vi "Transparent_VI.vi"(5 "Error_In":errorcluster) -> (19 "Error_Out":errorcluster)   [LabVIEW 2023]
doc: "Used to Popup in background for better UI and UX"
uses:
  Controls/UE_Driver_Operation_Select.ctl
types:
  T1 = typedef "UE_Driver_Operation_Select.ctl" = enum16{"Create_UE", "Get_Refnum", "Generate_UE", "Destroy_UE"}
  T2 = enum32{"Invalid", "Standard", "Closed", "Hidden", "Minimized", "Maximized"}
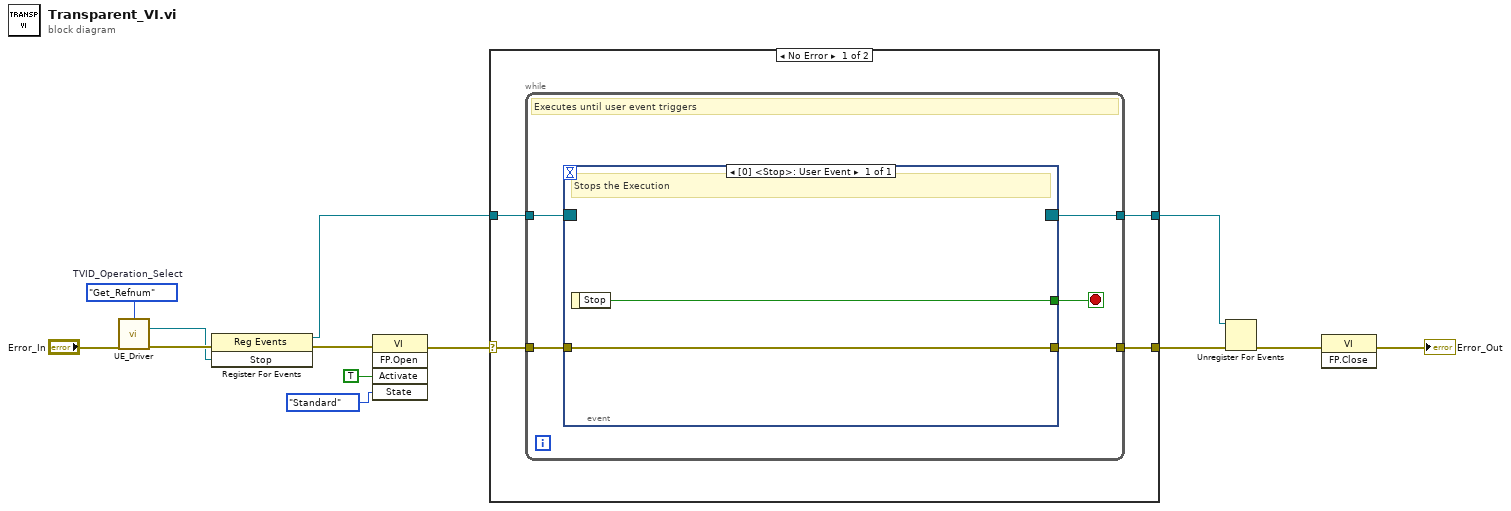
[diagram p0: block diagram]
diagram:
  w6 = UE_Driver_Operation_Select."Get_Refnum"  # TVID_Operation_Select
  n1 = call "UE_Driver.vi"("TVID_Operation_Select"=w6, "Error_In"="Error_In") -> ("Stop"=w4:refnum<user-event>, "Error_Out"=w7:errorcluster)  [unwired: 11 in, 1 out]
  n2 = register-events(error in=w7, w4) -> (reference out=w3:refnum<event-registration>, error out=w5:errorcluster)  [unwired: 1 in]
  n3 = invoke class="VI" method="FP.Open"(error in=w5, "Activate"=TRUE ("Activate?"), "State"=T2."Standard") -> (error out=w12:errorcluster)  [unwired: 2 in, 4 out]
  n4 = case shown="No Error" w12 {
    selector: w12 -> [w17 w26]
    tunnel: [w16 w26] -> w13
    tunnel: w3 -> [w15 w25]
    tunnel: [w14 w25] -> w1
    frame No Error {
      n5 = while {
        tunnel: w17 -> [w21]
        tunnel: [w20] -> w16
        tunnel: w15 -> [w19]
        tunnel: [w18] -> w14
        stop <- w22 stop-if-true
        # "Executes until user event triggers"
        n6 = event shown="[0] <Stop>: User Event" {
          selector: w19 -> [_]
          dyn-events: [_] -> w18
          timeout: _ -> [_]
          tunnel: [w23] -> w22
          tunnel: w21 -> [w24]
          tunnel: [w24] -> w20
          event User Event {
            # "Stops the Execution"
            n7 = event-data() -> ("Stop"=w23:bool)  [unwired: 1 in]
          }
        }
      }
    }
    frame Error {
    }
  }
  n8 = Unregister For Events(event registration refnum=w1, error in=w13) -> (error out=w2:errorcluster)
  n9 = invoke class="VI" method="FP.Close"(error in=w2) -> (error out=→"Error_Out":errorcluster)  [unwired: 2 in, 2 out]
